vi "Gainadjustment.vi"(1 "Gain":dbl[](array[numeric])=[100.0, 100.0, 100.0, 100.0, 100.0, 100.0, 100.0, 100.0, 100.0, 100.0, 100.0, 100.0, 100.0, 100.0, 100.0, 100.0, 100.0, 100.0, 100.0, 100.0, 100.0, 100.0, 100.0, 100.0, 100.0, 100.0, 100.0, 100.0, 100.0, 100.0, 100.0], 2 "CH 0 Data Path (.csv)":path) -> (0 "Adjusted gain":dbl[](array[numeric])=[99.5, 99.5, 99.5, 99.5, 99.5, 99.5, 99.5, 99.5, 99.5, 99.5, 99.5, 99.5, 99.5, 99.5, 99.5, 99.5, 99.5, 99.5, 99.5, 99.5, 99.5, 99.5, 99.5, 99.5, 99.5, 99.5, 99.5, 99.5, 99.5, 99.5, 99.5])   [LabVIEW 2020]
uses:
  <vilib>/Utility/file.llb/Read From Spreadsheet File (DBL).vi
  <vilib>/gmath/NI_Gmath.lvlib
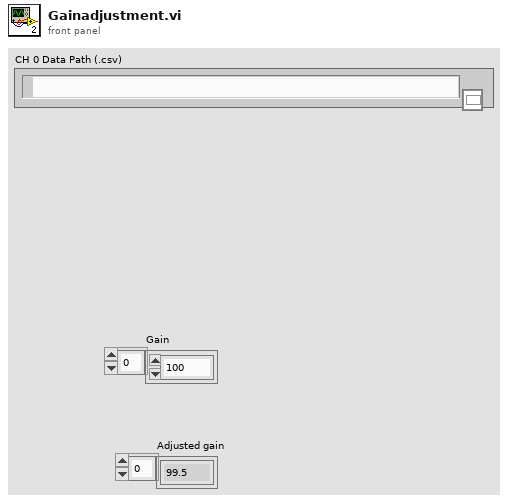
[diagram p1: front panel]
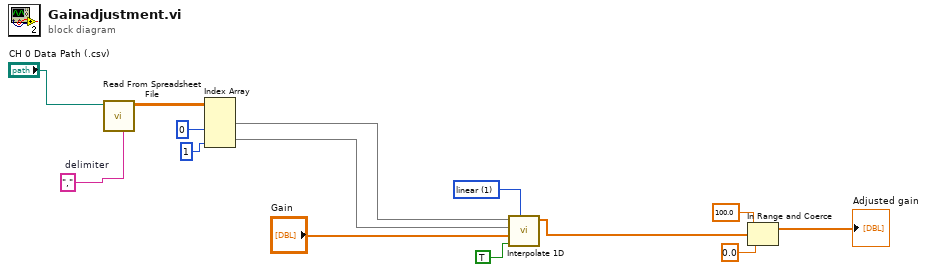
[diagram p0: block diagram]
diagram:
  w10 = 1 items=["nearest", "linear", "spline", "cubic Hermite", "Lagrange"] ("method")
  w13 = ","  # delimiter
  n1 = call-poly <vilib>:"Read From Spreadsheet File.vi"("delimiter (\\t)"=w13, "file path (dialog if empty)"="CH 0 Data Path (.csv)") -> ("all rows"=w12:dbl[][])  [unwired: 5 in, 4 out]
  n2 = Index Array(array=w12, index (col) #1=0, index (col) #2=1) -> (element #1=w2:dbl[], element #2=w1:dbl[])  [unwired: 2 in]
  n3 = call <vilib>:"Interpolate 1D.vi"("method"=w10, "X is monotonic"=TRUE, "xi"="Gain", "X"=w1, "Y"=w2) -> ("yi"=w8:dbl[])  [unwired: 4 in, 2 out]
  n4 = In Range and Coerce(upper limit=100.0, x=w8, lower limit=0.0) -> (coerced(x)=→"Adjusted gain":dbl[])  [unwired: 1 out]
